vi "DB_PRINCIPAL.vi"(8 "error in (no error)":errorcluster, 10 "password":string, 11 "userID":string) -> (0 "error out":errorcluster, 3 "connection reference":T1)   [LabVIEW 2019, in "DB_VENDING MACHINE.lvlib"]
doc: "Aquí se realiza la conexión a nuestra base de datos"
uses:
  DB_VENDING MACHINE.lvlib
  <vilib>/addons/database/Connection.llb/Conn ObjectReference.ctl
  <vilib>/addons/database/Connection.llb/DB Tools Open Connec (Path).vi
  <vilib>/addons/database/NI_Database_API.lvlib
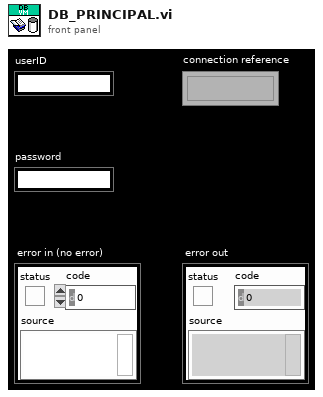
[diagram p1: front panel]
types:
  T1 = typedef "NI_Database_API.lvlib/Conn ObjectReference.ctl" = refnum<k1>
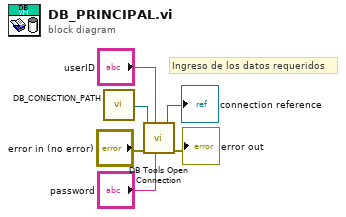
[diagram p0: block diagram]
diagram:
  # "Ingreso de los datos requeridos"
  n1 = call "DB_CONECTION_PATH.vi"() -> ("Conection path"=w5:path)  [unwired: 11 in]
  n2 = call-poly <vilib>:"DB Tools Open Connection.vi"("password"="password", "userID"="userID", "error in (no error)"="error in (no error)", "connection information"=w5) -> ("error out"=→"error out":errorcluster, "connection reference"=→"connection reference":T1)  [unwired: 4 in]
